vi "Play_SoundFile.vi"(8 "error in (no error)":errorcluster, 11 "File Path In":path) -> (0 "error out":errorcluster, 3 "File Path Out":path)   [LabVIEW 2018, in "MerriamWebsterJSON.lvlib"]
uses:
  MerriamWebsterJSON.lvlib
  <vilib>/sound2/lvsound2.llb/Sound Data Format.ctl
  74b8f871-41e0-43b4-bfdd-f093a6785aa0.vi
  <vilib>/sound2/lvsound2.llb/Sound File Read Open.vi
  <vilib>/sound2/lvsound2.llb/Sound File Read (DBL).vi
  <vilib>/sound2/lvsound2.llb/Sound Output Write (DBL).vi
panel:
  out "Sound":waveform(dbl)[](graph)
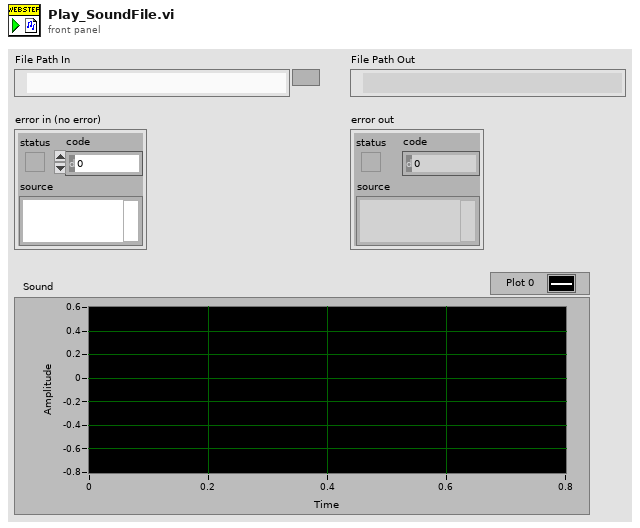
[diagram p1: front panel]
types:
  T1 = typedef "Sound Data Format.ctl" = cluster{"sample rate (S/s)":dbl, "number of channels":i32, "bits per sample":i32}
  T2 = typedef "Sound File Refnum.ctl" = refnum<file>
  T3 = typedef "Sound Output Task ID.ctl" = u32
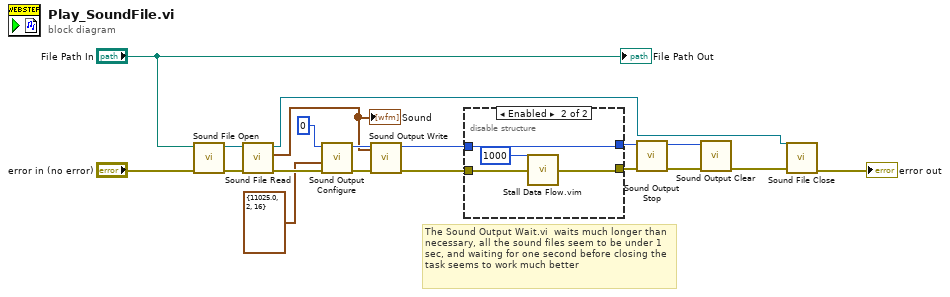
[diagram p0: block diagram]
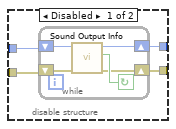
[diagram p2: hidden frame]
diagram:
  # "The Sound Output Wait.vi  waits much longer than necessary, all the sound files seem to be under 1 sec, and waiting for one second before closing the task seems to work much better"
  n1 = call-poly <vilib>:"Sound File Open.vi"("error in (no error)"="error in (no error)", "path"="File Path In") -> ("error out"=w17:errorcluster, "sound file refnum"=w19:T2)  [unwired: 8 in]
  n2 = call-poly <vilib>:"Sound File Read.vi"("error in (no error)"=w17, "sound file refnum"=w19) -> ("error out"=w15:errorcluster, "data"=w1:waveform(dbl)[], "sound file refnum out"=w10:T2)  [unwired: 5 in, 2 out]
  "Sound" <- w1
  n3 = call <vilib>:"Sound Output Configure.vi"("error in (no error)"=w15, "sound format"=T1 {"sample rate (S/s)"=11025.0, "number of channels"=2, "bits per sample"=16}, "device ID"=u32 0) -> ("error out"=w8:errorcluster, "task ID"=w14:T3)  [unwired: 7 in]
  n4 = call-poly <vilib>:"Sound Output Write.vi"("error in (no error)"=w8, "data"=w1, "task ID"=w14) -> ("error out"=w4:errorcluster, "task ID out"=w5:T3)  [unwired: 7 in]
  n5 = disable-structure shown="Enabled" {
    disable-tunnel: w5 -> [w23 w32]
    disable-tunnel: w4 -> [w22 w31]
    disable-tunnel: [w21 w32] -> w3
    disable-tunnel: [w20 w30] -> w2
    frame Disabled {
      n6 = while {
        shift-right: [w25] -> w21
        shift-left: w23 -> [w27]
        shift-right: [w24] -> w20
        shift-left: w22 -> [w28]
        stop <- w26 continue-if-true
        n7 = call <vilib>:"Sound Output Info.vi"("error in (no error)"=w28, "task ID"=w27) -> ("error out"=w24:errorcluster, "is playing?"=w26:bool, "task ID out"=w25:T3)  [unwired: 6 in, 1 out]
      }
    }
    frame Enabled {
      n8 = call "Stall Data Flow.vim"("value in"=w31, "milliseconds to wait"=u32 1000) -> ("value out"=w30:errorcluster)  [unwired: 1 out]
    }
  }
  n9 = call <vilib>:"Sound Output Stop.vi"("error in (no error)"=w2, "task ID"=w3) -> ("error out"=w12:errorcluster, "task ID out"=w13:T3)  [unwired: 8 in]
  n10 = call <vilib>:"Sound Output Clear.vi"("error in (no error)"=w12, "task ID"=w13) -> ("error out"=w11:errorcluster)  [unwired: 9 in]
  n11 = call <vilib>:"Sound File Close.vi"("error in (no error)"=w11, "sound file refnum"=w10) -> ("error out"=→"error out":errorcluster)  [unwired: 9 in]
  "File Path Out" <- "File Path In"
